vi "Create 2 In 2 Out Channel Resources.vi"(0 "common resources":T18={"sync pulse resources"={"sync pulse destination terminal"="", "sync100"="", "sync pulse source terminal"="", "imported sync pulse register"="", "generate sync pulse handshake"="", "enable sync pulse register"="", "sync pulse clock"=""}, "serial channel resources"={"sc 0"={"completed frames register"=""}, "sc 1"={"completed frames register"=""}, "sc 2"={"completed frames register"=""}, "sc 3"={"completed frames register"=""}, "sc 4"={"completed frames register"=""}, "sc 5"={"completed frames register"=""}, "sc 6"={"completed frames register"=""}, "sc 7"={"completed frames register"=""}}, "dram manager 0"={"DRAM class"=refnum, "process clock"="", "registers"={"configuration"={"write time slice"="", "request time slice"="", "DRAM arbiter config"="", "partition config"=""}, "reset"={"handshake"={"start.go"="", "start.go rcvd"="", "done.go"="", "done.go rcvd"=""}, "process"={"in"="", "out"=""}, "write"={"in"="", "out 0"="", "out 1"="", "out 2"="", "out 3"=""}, "read"={"in"="", "out 0"="", "out 1"="", "out 2"="", "out 3"=""}}, "status"={"partition full"=""}}, "FIFOs"={"write data"={"FIFO 0"="", "FIFO 1"="", "FIFO 2"="", "FIFO 3"=""}, "request metadata"={"FIFO"=""}, "read data VOQ"={"FIFO 0"="", "FIFO 1"="", "FIFO 2"="", "FIFO 3"=""}, "read data"={"FIFO 0"="", "FIFO 1"="", "FIFO 2"="", "FIFO 3"=""}}, "num active streams"=0.0, "max open read requests"=256}, "dram manager 1"={"DRAM class"=refnum, "process clock"="", "registers"={"configuration"={"write time slice"="", "request time slice"="", "DRAM arbiter config"="", "partition config"=""}, "reset"={"handshake"={"start.go"="", "start.go rcvd"="", "done.go"="", "done.go rcvd"=""}, "process"={"in"="", "out"=""}, "write"={"in"="", "out 0"="", "out 1"="", "out 2"="", "out 3"=""}, "read"={"in"="", "out 0"="", "out 1"="", "out 2"="", "out 3"=""}}, "status"={"partition full"=""}}, "FIFOs"={"write data"={"FIFO 0"="", "FIFO 1"="", "FIFO 2"="", "FIFO 3"=""}, "request metadata"={"FIFO"=""}, "read data VOQ"={"FIFO 0"="", "FIFO 1"="", "FIFO 2"="", "FIFO 3"=""}, "read data"={"FIFO 0"="", "FIFO 1"="", "FIFO 2"="", "FIFO 3"=""}}, "num active streams"=0.0, "max open read requests"=256}}, 5 "dram partition configs":T22[](array[typedef])=[{"first address"=0, "last address"=0}, {"first address"=0, "last address"=0}, {"first address"=0, "last address"=0}, {"first address"=0, "last address"=0}, {"first address"=0, "last address"=0}, {"first address"=0, "last address"=0}, {"first address"=0, "last address"=0}, {"first address"=0, "last address"=0}]) -> (4 "channel resources":T1)   [LabVIEW 2020, in "GettingStarted_Acq_Tap_148X_FPGA.lvlib"]
uses:
  GettingStarted_Acq_Tap_148X_FPGA.lvlib
  <instrlib>/FlexRIO/CSI-2/v2/FPGA/DRAM Manager/Public/Partition Range.ctl
  Common/Types/Common Resources.ctl
  <instrlib>/_niInstr/Memory/v1/FPGA/DRAM/niInstr Memory DRAM v1 FPGA.lvclass
  <instrlib>/FlexRIO/CSI-2/v2/FPGA/Types/Sync Pulse Resources.ctl
  Common/Types/Serial Channel Resources.ctl
  Common/Types/Single Serial Channel Resources.ctl
  <instrlib>/FlexRIO/CSI-2/v2/FPGA/DRAM Manager/Private/DRAM Manager.ctl
  <instrlib>/FlexRIO/CSI-2/v2/FPGA/DRAM Manager/Private/Common/DRAM Manager Registers.ctl
  <instrlib>/FlexRIO/CSI-2/v2/FPGA/DRAM Manager/Private/Common/Handshake Registers.ctl
  <instrlib>/FlexRIO/CSI-2/v2/FPGA/DRAM Manager/Private/Common/DRAM Manager FIFOs.ctl
  <instrlib>/FlexRIO/CSI-2/v2/FPGA/DRAM Manager/Private/Common/Write Data FIFO Ref.ctl
  <instrlib>/FlexRIO/CSI-2/v2/FPGA/DRAM Manager/Private/Common/Read Request Metadata FIFO Ref.ctl
  <instrlib>/FlexRIO/CSI-2/v2/FPGA/DRAM Manager/Private/Common/Read Data FIFO Ref.ctl
  Types/2 In 2 Out Channel Resources.ctl
  Types/Serial Input Channel Resources.ctl
  Types/Serial Input Channel IO.ctl
  Types/Serial Input Channel IO 32b.ctl
  Types/Serial Input Channel IO 64b.ctl
  Common/Types/I2C IO.ctl
  Types/Serial Ouput Channel Resources.ctl
  Common/Types/Serial Output Channel IO.ctl
  Common/Types/Serial Output Channel IO 32b.ctl
  Common/Types/Serial Output Channel IO 64b.ctl
  <instrlib>/FlexRIO/CSI-2/v2/FPGA/DRAM Manager/DRAM Manager v2.lvlib
  Common/GettingStarted_Common_148X_FPGA.lvlib
  <instrlib>/FlexRIO/CSI-2/v2/FPGA/NI CSI-2 API FPGA v2.lvlib
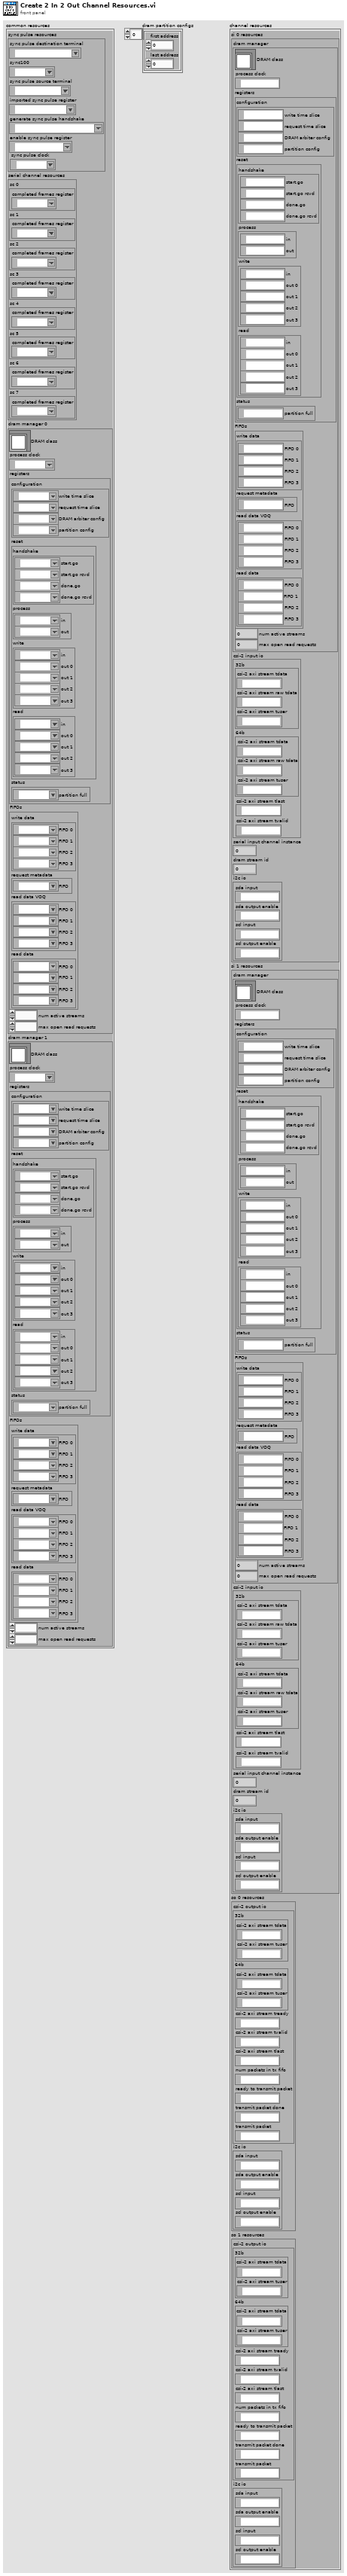
[diagram p1: front panel]
types:
  T1 = typedef "GettingStarted_Acq_Tap_148X_FPGA.lvlib/2 In 2 Out Channel Resources.ctl" = cluster{"si 0 resources":T2, "si 1 resources":T2, "so 0 resources":T14, "so 1 resources":T14}
  T2 = typedef "GettingStarted_Acq_Tap_148X_FPGA.lvlib/Serial Input Channel Resources.ctl" = cluster{"dram manager":T3, "csi-2 input io":T10, "serial input channel instance":u8, "dram stream id":fxp<+,2,2>, "i2c io":T13}
  T3 = typedef "DRAM Manager v2.lvlib/DRAM Manager.ctl" = cluster{"DRAM class":refnum<class "niInstr Memory DRAM v1 FPGA.lvclass">, "process clock":refnum<k21>, "registers":T4, "FIFOs":T6, "num active streams":fxp<+,3,3>, "max open read requests":u16}
  T4 = typedef "DRAM Manager v2.lvlib/DRAM Manager Registers.ctl" = cluster{"configuration":cluster{"write time slice":refnum<k21>, "request time slice":refnum<k21>, "DRAM arbiter config":refnum<k21>, "partition config":refnum<k21>}, "reset":cluster{"handshake":T5, "process":cluster{"in":refnum<k21>, "out":refnum<k21>}, "write":cluster{"in":refnum<k21>, "out 0":refnum<k21>, "out 1":refnum<k21>, "out 2":refnum<k21>, "out 3":refnum<k21>}, "read":cluster{"in":refnum<k21>, "out 0":refnum<k21>, "out 1":refnum<k21>, "out 2":refnum<k21>, "out 3":refnum<k21>}}, "status":cluster{"partition full":refnum<k21>}}
  T5 = typedef "DRAM Manager v2.lvlib/Handshake Registers.ctl" = cluster{"start.go":refnum<k21>, "start.go rcvd":refnum<k21>, "done.go":refnum<k21>, "done.go rcvd":refnum<k21>}
  T6 = typedef "DRAM Manager v2.lvlib/DRAM Manager FIFOs.ctl" = cluster{"write data":cluster{"FIFO 0":T7, "FIFO 1":T7, "FIFO 2":T7, "FIFO 3":T7}, "request metadata":cluster{"FIFO":T8}, "read data VOQ":cluster{"FIFO 0":T9, "FIFO 1":T9, "FIFO 2":T9, "FIFO 3":T9}, "read data":cluster{"FIFO 0":T9, "FIFO 1":T9, "FIFO 2":T9, "FIFO 3":T9}}
  T7 = typedef "DRAM Manager v2.lvlib/Write Data FIFO Ref.ctl" = refnum<k21>
  T8 = typedef "DRAM Manager v2.lvlib/Read Request Metadata FIFO Ref.ctl" = refnum<k21>
  T9 = typedef "DRAM Manager v2.lvlib/Read Data FIFO Ref.ctl" = refnum<k21>
  T10 = typedef "GettingStarted_Acq_Tap_148X_FPGA.lvlib/Serial Input Channel IO.ctl" = cluster{"32b":T11, "64b":T12, "csi-2 axi stream tlast":refnum<k21>, "csi-2 axi stream tvalid":refnum<k21>}
  T11 = typedef "GettingStarted_Acq_Tap_148X_FPGA.lvlib/Serial Input Channel IO 32b.ctl" = cluster{"csi-2 axi stream tdata":refnum<k21>, "csi-2 axi stream raw tdata":refnum<k21>, "csi-2 axi stream tuser":refnum<k21>}
  T12 = typedef "GettingStarted_Acq_Tap_148X_FPGA.lvlib/Serial Input Channel IO 64b.ctl" = cluster{"csi-2 axi stream tdata":refnum<k21>, "csi-2 axi stream raw tdata":refnum<k21>, "csi-2 axi stream tuser":refnum<k21>}
  T13 = typedef "GettingStarted_Common_148X_FPGA.lvlib/I2C IO.ctl" = cluster{"sda input":refnum<k21>, "sda output enable":refnum<k21>, "scl input":refnum<k21>, "scl output enable":refnum<k21>}
  T14 = typedef "GettingStarted_Acq_Tap_148X_FPGA.lvlib/Serial Ouput Channel Resources.ctl" = cluster{"csi-2 output io":T15, "i2c io":T13}
  T15 = typedef "GettingStarted_Common_148X_FPGA.lvlib/Serial Output Channel IO.ctl" = cluster{"32b":T16, "64b":T17, "csi-2 axi stream tready":refnum<k21>, "csi-2 axi stream tvalid":refnum<k21>, "csi-2 axi stream tlast":refnum<k21>, "num packets in tx fifo":refnum<k21>, "ready to transmit packet":refnum<k21>, "transmit packet done":refnum<k21>, "transmit packet":refnum<k21>}
  T16 = typedef "GettingStarted_Common_148X_FPGA.lvlib/Serial Output Channel IO 32b.ctl" = cluster{"csi-2 axi stream tdata":refnum<k21>, "csi-2 axi stream tuser":refnum<k21>}
  T17 = typedef "GettingStarted_Common_148X_FPGA.lvlib/Serial Output Channel IO 64b.ctl" = cluster{"csi-2 axi stream tdata":refnum<k21>, "csi-2 axi stream tuser":refnum<k21>}
  T18 = typedef "GettingStarted_Common_148X_FPGA.lvlib/Common Resources.ctl" = cluster{"sync pulse resources":T19, "serial channel resources":T20, "dram manager 0":T3, "dram manager 1":T3}
  T19 = typedef "NI CSI-2 API FPGA v2.lvlib/Sync Pulse Resources.ctl" = cluster{"sync pulse destination terminal":refnum<k21>, "sync100":refnum<k21>, "sync pulse source terminal":refnum<k21>, "imported sync pulse register":refnum<k21>, "generate sync pulse handshake":refnum<k21>, "enable sync pulse register":refnum<k21>, "sync pulse clock":refnum<k21>}
  T20 = typedef "GettingStarted_Common_148X_FPGA.lvlib/Serial Channel Resources.ctl" = cluster{"sc 0":T21, "sc 1":T21, "sc 2":T21, "sc 3":T21, "sc 4":T21, "sc 5":T21, "sc 6":T21, "sc 7":T21}
  T21 = typedef "GettingStarted_Common_148X_FPGA.lvlib/Single Serial Channel Resources.ctl" = cluster{"completed frames register":refnum<k21>}
  T22 = typedef "DRAM Manager v2.lvlib/Partition Range.ctl" = cluster{"first address":u32, "last address":u32}
  T23 = cluster{"serial input 0 csi-2 io":T10, "serial input 1 csi-2 io":T10}
  T24 = cluster{"serial input 0 i2c io":T13, "serial input 1 i2c io":T13}
  T25 = cluster{"serial output 0 io":T15, "serial output 1 io":T15}
  T26 = cluster{"serial output 0 i2c io":T13, "serial output 1 i2c io":T13}
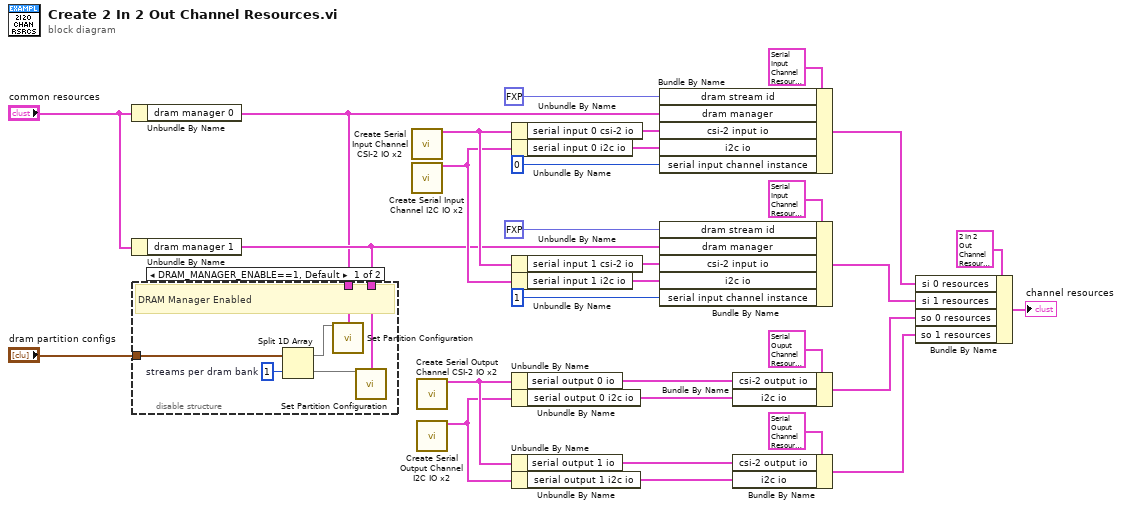
[diagram p0: block diagram]
diagram:
  n1 = Unbundle By Name("common resources") -> ("dram manager 0"=w1:T3)
  n2 = Unbundle By Name("common resources") -> ("dram manager 1"=w2:T3)
  n3 = disable-structure shown="DRAM_MANAGER_ENABLE==1, Default" {
    disable-tunnel: "dram partition configs" -> [w35 _]
    disable-tunnel: w2 -> [w32 _]
    disable-tunnel: w1 -> [w31 _]
    frame condition #0 (active) {
      w36 = 1  # streams per dram bank
      # "DRAM Manager Enabled"
      n4 = Split 1D Array(array=w35, index=w36) -> (first subarray=w34:T22[], second subarray=w33:T22[])
      n5 = call <instrlib>:"Set Partition Configuration.vi"("partition config"=w34, "DRAM manager"=w31) -> ()  [unwired: 14 in]
      n6 = call <instrlib>:"Set Partition Configuration.vi"("partition config"=w33, "DRAM manager"=w32) -> ()  [unwired: 14 in]
    }
    frame condition #1 {
      # "DRAM Manager Disabled"
    }
  }
  n7 = call "Create Serial Input Channel CSI-2 IO x2.vi"() -> ("serial input csi-2 io x2"=w17:T23)  [unwired: 15 in]
  n8 = call "Create Serial Input Channel I2C IO x2.vi"() -> ("serial input channel i2c io x2"=w8:T24)  [unwired: 15 in]
  n9 = call "Create Serial Output Channel CSI-2 IO x2.vi"() -> ("serial output channel csi-2 io x2"=w14:T25)  [unwired: 15 in]
  n10 = call "Create Serial Output Channel I2C IO x2.vi"() -> ("serial output channel i2c io x2"=w11:T26)  [unwired: 15 in]
  n11 = Unbundle By Name(w17) -> ("serial input 0 csi-2 io"=w19:T10)
  n12 = Unbundle By Name(w8) -> ("serial input 0 i2c io"=w9:T13)
  n13 = Unbundle By Name(w17) -> ("serial input 1 csi-2 io"=w18:T10)
  n14 = Unbundle By Name(w8) -> ("serial input 1 i2c io"=w10:T13)
  n15 = Unbundle By Name(w14) -> ("serial output 0 io"=w16:T15)
  n16 = Unbundle By Name(w11) -> ("serial output 0 i2c io"=w13:T13)
  n17 = Unbundle By Name(w14) -> ("serial output 1 io"=w15:T15)
  n18 = Unbundle By Name(w11) -> ("serial output 1 i2c io"=w12:T13)
  n19 = Bundle By Name(cluster=T2 {"dram manager"={"DRAM class"=refnum, "process clock"="", "registers"={"configuration"={"write time slice"="", "request time slice"="", "DRAM arbiter config"="", "partition config"=""}, "reset"={"handshake"={"start.go"="", "start.go rcvd"="", "done.go"="", "done.go rcvd"=""}, "process"={"in"="", "out"=""}, "write"={"in"="", "out 0"="", "out 1"="", "out 2"="", "out 3"=""}, "read"={"in"="", "out 0"="", "out 1"="", "out 2"="", "out 3"=""}}, "status"={"partition full"=""}}, "FIFOs"={"write data"={"FIFO 0"="", "FIFO 1"="", "FIFO 2"="", "FIFO 3"=""}, "request metadata"={"FIFO"=""}, "read data VOQ"={"FIFO 0"="", "FIFO 1"="", "FIFO 2"="", "FIFO 3"=""}, "read data"={"FIFO 0"="", "FIFO 1"="", "FIFO 2"="", "FIFO 3"=""}}, "num active streams"=0.0, "max open read requests"=0}, "csi-2 input io"={"32b"={"csi-2 axi stream tdata"="", "csi-2 axi stream raw tdata"="", "csi-2 axi stream tuser"=""}, "64b"={"csi-2 axi stream tdata"="", "csi-2 axi stream raw tdata"="", "csi-2 axi stream tuser"=""}, "csi-2 axi stream tlast"="", "csi-2 axi stream tvalid"=""}, "serial input channel instance"=0, "dram stream id"=0.0, "i2c io"={"sda input"="", "sda output enable"="", "scl input"="", "scl output enable"=""}} ("si 0 resources"), "dram stream id"=fxp<+,2,2> 0.0, "dram manager"=w1, "csi-2 input io"=w19, "i2c io"=w9, "serial input channel instance"=u8 0) -> (w30:T2)
  n20 = Bundle By Name(cluster=T2 {"dram manager"={"DRAM class"=refnum, "process clock"="", "registers"={"configuration"={"write time slice"="", "request time slice"="", "DRAM arbiter config"="", "partition config"=""}, "reset"={"handshake"={"start.go"="", "start.go rcvd"="", "done.go"="", "done.go rcvd"=""}, "process"={"in"="", "out"=""}, "write"={"in"="", "out 0"="", "out 1"="", "out 2"="", "out 3"=""}, "read"={"in"="", "out 0"="", "out 1"="", "out 2"="", "out 3"=""}}, "status"={"partition full"=""}}, "FIFOs"={"write data"={"FIFO 0"="", "FIFO 1"="", "FIFO 2"="", "FIFO 3"=""}, "request metadata"={"FIFO"=""}, "read data VOQ"={"FIFO 0"="", "FIFO 1"="", "FIFO 2"="", "FIFO 3"=""}, "read data"={"FIFO 0"="", "FIFO 1"="", "FIFO 2"="", "FIFO 3"=""}}, "num active streams"=0.0, "max open read requests"=0}, "csi-2 input io"={"32b"={"csi-2 axi stream tdata"="", "csi-2 axi stream raw tdata"="", "csi-2 axi stream tuser"=""}, "64b"={"csi-2 axi stream tdata"="", "csi-2 axi stream raw tdata"="", "csi-2 axi stream tuser"=""}, "csi-2 axi stream tlast"="", "csi-2 axi stream tvalid"=""}, "serial input channel instance"=0, "dram stream id"=0.0, "i2c io"={"sda input"="", "sda output enable"="", "scl input"="", "scl output enable"=""}} ("si 0 resources"), "dram stream id"=fxp<+,2,2> 0.0, "dram manager"=w2, "csi-2 input io"=w18, "i2c io"=w10, "serial input channel instance"=u8 1) -> (w29:T2)
  n21 = Bundle By Name(cluster=T14 {"csi-2 output io"={"32b"={"csi-2 axi stream tdata"="", "csi-2 axi stream tuser"=""}, "64b"={"csi-2 axi stream tdata"="", "csi-2 axi stream tuser"=""}, "csi-2 axi stream tready"="", "csi-2 axi stream tvalid"="", "csi-2 axi stream tlast"="", "num packets in tx fifo"="", "ready to transmit packet"="", "transmit packet done"="", "transmit packet"=""}, "i2c io"={"sda input"="", "sda output enable"="", "scl input"="", "scl output enable"=""}} ("so 0 resources"), "csi-2 output io"=w16, "i2c io"=w13) -> (w4:T14)
  n22 = Bundle By Name(cluster=T14 {"csi-2 output io"={"32b"={"csi-2 axi stream tdata"="", "csi-2 axi stream tuser"=""}, "64b"={"csi-2 axi stream tdata"="", "csi-2 axi stream tuser"=""}, "csi-2 axi stream tready"="", "csi-2 axi stream tvalid"="", "csi-2 axi stream tlast"="", "num packets in tx fifo"="", "ready to transmit packet"="", "transmit packet done"="", "transmit packet"=""}, "i2c io"={"sda input"="", "sda output enable"="", "scl input"="", "scl output enable"=""}} ("so 0 resources"), "csi-2 output io"=w15, "i2c io"=w12) -> (w3:T14)
  n23 = Bundle By Name(cluster=T1 {"si 0 resources"={"dram manager"={"DRAM class"=refnum, "process clock"="", "registers"={"configuration"={"write time slice"="", "request time slice"="", "DRAM arbiter config"="", "partition config"=""}, "reset"={"handshake"={"start.go"="", "start.go rcvd"="", "done.go"="", "done.go rcvd"=""}, "process"={"in"="", "out"=""}, "write"={"in"="", "out 0"="", "out 1"="", "out 2"="", "out 3"=""}, "read"={"in"="", "out 0"="", "out 1"="", "out 2"="", "out 3"=""}}, "status"={"partition full"=""}}, "FIFOs"={"write data"={"FIFO 0"="", "FIFO 1"="", "FIFO 2"="", "FIFO 3"=""}, "request metadata"={"FIFO"=""}, "read data VOQ"={"FIFO 0"="", "FIFO 1"="", "FIFO 2"="", "FIFO 3"=""}, "read data"={"FIFO 0"="", "FIFO 1"="", "FIFO 2"="", "FIFO 3"=""}}, "num active streams"=0.0, "max open read requests"=0}, "csi-2 input io"={"32b"={"csi-2 axi stream tdata"="", "csi-2 axi stream raw tdata"="", "csi-2 axi stream tuser"=""}, "64b"={"csi-2 axi stream tdata"="", "csi-2 axi stream raw tdata"="", "csi-2 axi stream tuser"=""}, "csi-2 axi stream tlast"="", "csi-2 axi stream tvalid"=""}, "serial input channel instance"=0, "dram stream id"=0.0, "i2c io"={"sda input"="", "sda output enable"="", "scl input"="", "scl output enable"=""}}, "si 1 resources"={"dram manager"={"DRAM class"=refnum, "process clock"="", "registers"={"configuration"={"write time slice"="", "request time slice"="", "DRAM arbiter config"="", "partition config"=""}, "reset"={"handshake"={"start.go"="", "start.go rcvd"="", "done.go"="", "done.go rcvd"=""}, "process"={"in"="", "out"=""}, "write"={"in"="", "out 0"="", "out 1"="", "out 2"="", "out 3"=""}, "read"={"in"="", "out 0"="", "out 1"="", "out 2"="", "out 3"=""}}, "status"={"partition full"=""}}, "FIFOs"={"write data"={"FIFO 0"="", "FIFO 1"="", "FIFO 2"="", "FIFO 3"=""}, "request metadata"={"FIFO"=""}, "read data VOQ"={"FIFO 0"="", "FIFO 1"="", "FIFO 2"="", "FIFO 3"=""}, "read data"={"FIFO 0"="", "FIFO 1"="", "FIFO 2"="", "FIFO 3"=""}}, "num active streams"=0.0, "max open read requests"=0}, "csi-2 input io"={"32b"={"csi-2 axi stream tdata"="", "csi-2 axi stream raw tdata"="", "csi-2 axi stream tuser"=""}, "64b"={"csi-2 axi stream tdata"="", "csi-2 axi stream raw tdata"="", "csi-2 axi stream tuser"=""}, "csi-2 axi stream tlast"="", "csi-2 axi stream tvalid"=""}, "serial input channel instance"=0, "dram stream id"=0.0, "i2c io"={"sda input"="", "sda output enable"="", "scl input"="", "scl output enable"=""}}, "so 0 resources"={"csi-2 output io"={"32b"={"csi-2 axi stream tdata"="", "csi-2 axi stream tuser"=""}, "64b"={"csi-2 axi stream tdata"="", "csi-2 axi stream tuser"=""}, "csi-2 axi stream tready"="", "csi-2 axi stream tvalid"="", "csi-2 axi stream tlast"="", "num packets in tx fifo"="", "ready to transmit packet"="", "transmit packet done"="", "transmit packet"=""}, "i2c io"={"sda input"="", "sda output enable"="", "scl input"="", "scl output enable"=""}}, "so 1 resources"={"csi-2 output io"={"32b"={"csi-2 axi stream tdata"="", "csi-2 axi stream tuser"=""}, "64b"={"csi-2 axi stream tdata"="", "csi-2 axi stream tuser"=""}, "csi-2 axi stream tready"="", "csi-2 axi stream tvalid"="", "csi-2 axi stream tlast"="", "num packets in tx fifo"="", "ready to transmit packet"="", "transmit packet done"="", "transmit packet"=""}, "i2c io"={"sda input"="", "sda output enable"="", "scl input"="", "scl output enable"=""}}} ("2 in 2 out channel resources"), "si 0 resources"=w30, "si 1 resources"=w29, "so 0 resources"=w4, "so 1 resources"=w3) -> (→"channel resources":T1)
